vi "BPM.vi"(4 "error in (no error)":errorcluster, 6 "Max BPM Threshold":dbl, 7 "Time Stamp":timestamp) -> (0 "error out":errorcluster, 2 "BPM":dbl, 3 "Below MAX BPM Threshold?":bool)   [LabVIEW 2020]
doc: "Takes the <b>Time Stamp</b> of the last pulse and if the time stamp results in a BPM below <b>Max BPM Threshold</b> then the VI returns the <b>BPM</b> as well as the boolean <b>Below MAX BPM Threshold?</b>"
uses:
  <vilib>/Analysis/baseanly.llb/Mean (DBL).vi
  <vilib>/Analysis/NI_AALBase.lvlib
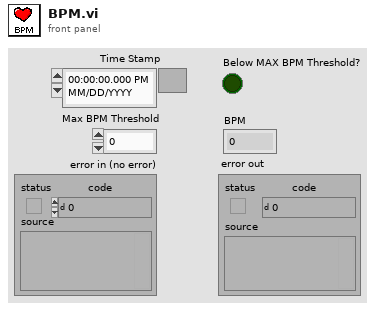
[diagram p1: front panel]
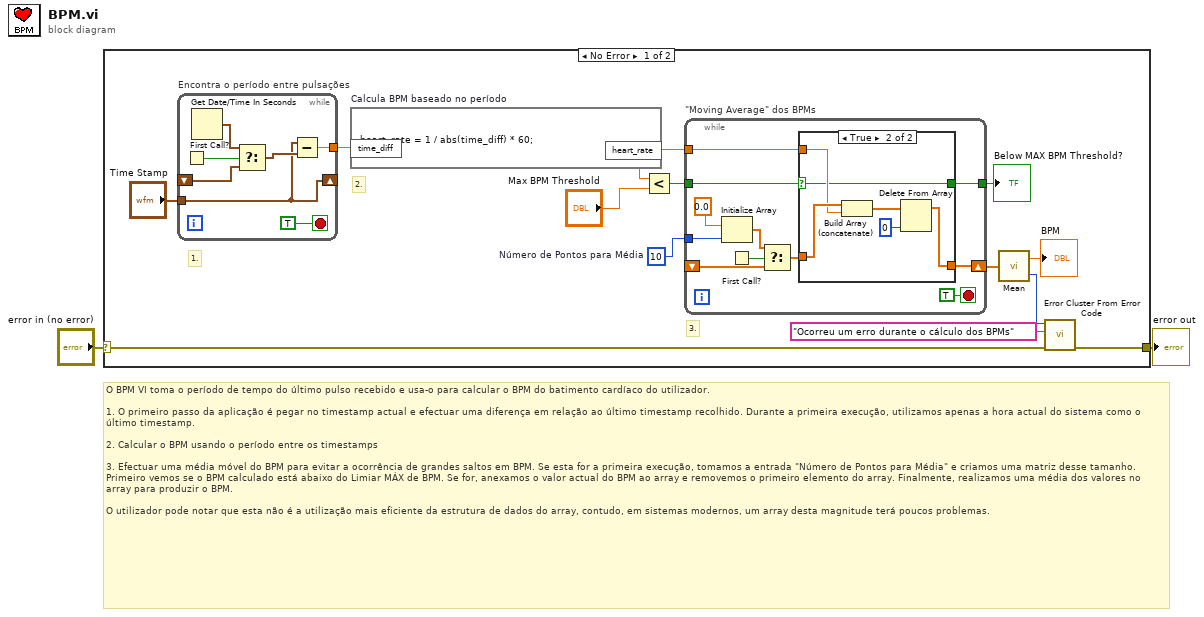
[diagram p0: block diagram]
diagram:
  # "O BPM VI toma o período de tempo do último pulso recebido e usa-o para calcular o BPM do batimento cardíaco do utilizador.\n\n1. O primeiro passo da aplicação é pegar no timestamp actual e efectuar uma diferença em relação ao último timestamp recolhido. Durante a primeira execução, utilizamos apenas a hora actual do sistema como o último timestamp.\n\n2. Calcular o BPM usando o período entre os timestamps\n\n3. Efectuar uma média móvel do BPM para evitar a ocorrência de grandes saltos em BPM. Se esta for a primeira execução, tomamos a entrada \"Número de Pontos para Média\" e criamos uma matriz desse tamanho. Primeiro vemos se o BPM calculado está abaixo do Limiar MÁX de BPM. Se for, anexamos o valor actual do BPM ao array e removemos o primeiro elemento do array. Finalmente, realizamos uma média dos valores no array para produzir o BPM.\n\nO utilizador pode notar que esta não é a utilização mais eficiente da estrutura de dados do array, contudo, em sistemas modernos, um array desta magnitude terá poucos problemas."
  n1 = case shown="No Error" "error in (no error)" {
    selector: "error in (no error)" -> [w8 w42]
    tunnel: [w9 w42] -> w1
    frame No Error {
      w3 = 10  # Número de Pontos para Média
      # "3."
      # "2."
      # "1."
      n2 = while "Encontra o período entre pulsações" {
        shift-right: [w17] -> _
        shift-left: _ -> [w19]
        tunnel: "Time Stamp" -> [w17]
        tunnel: [w16] -> w14
        stop <- TRUE stop-if-true
        n3 = First Call?() -> (First Call?: T/F=w20:bool)
        n4 = Get Date/Time In Seconds() -> (seconds since 1Jan1904=w21:timestamp)
        n5 = Select(t=w21, s=w20, f=w19) -> (s? t:f=w18:timestamp)
        n6 = Subtract(x=w17, y=w18) -> (x-y=w16:dbl)
      }
      n7 = formula code="heart_rate = 1 / abs(time_diff) * 60;" "Calcula BPM baseado no período"("time_diff"=w14) -> ("heart_rate"=w11:dbl)
      n8 = Less?(x=w11, y="Max BPM Threshold") -> (x < y?=w12:bool)
      n9 = while "\"Moving Average\" dos BPMs" {
        tunnel: w12 -> [w27]
        shift-right: [w26] -> w10
        shift-left: _ -> [w31]
        tunnel: w11 -> [w25]
        tunnel: [w24] -> w4
        tunnel: w3 -> [w23]
        stop <- TRUE stop-if-true
        n10 = Initialize Array(0.0 ("element"), w23) -> (w30:dbl[])
        n11 = First Call?() -> (First Call?: T/F=w32:bool)
        n12 = Select(t=w30, s=w32, f=w31) -> (s? t:f=w28:dbl[])
        n13 = case shown="True" w27 {
          selector: w27 -> [w34 w36]
          tunnel: w28 -> [w35 w41]
          tunnel: [w35 w37] -> w26
          tunnel: w25 -> [_ w40]
          tunnel: [w34 w36] -> w24
          frame False {
          }
          frame True {
            n14 = Build Array (concatenate)(w41, w40) -> (w39:dbl[])
            n15 = Delete From Array(array=w39, index=0) -> (array with subset deleted=w37:dbl[])  [unwired: 1 in, 1 out]
          }
        }
      }
      "Below MAX BPM Threshold?" <- w4
      n16 = call-poly <vilib>:"Mean.vi"("X"=w10) -> ("mean"=→"BPM":dbl, "error"=w6:i32)
      n17 = call <vilib>:"Error Cluster From Error Code.vi"("error in (no error)"=w8, "error message (\"\")"="Ocorreu um erro durante o cálculo dos BPMs" ("error message (\"\")"), "error code (0)"=w6) -> ("error out"=w9:errorcluster)  [unwired: 6 in]
    }
    frame Error {
    }
  }
  "error out" <- w1
